vi "RGBToIntensityGraph.vi"(3 "B Array":sgl[][](array[numeric])=array200x200[40000 elements], 4 "G Array":sgl[][](array[numeric])=array200x200[40000 elements], 5 "R Array":sgl[][](array[numeric])=array200x200[40000 elements]) -> (1 "2D Picture":picture)   [LabVIEW 2015]
uses:
  <vilib>/picture/picture.llb/Draw True-Color Pixmap.vi
panel:
  out "Intensity Graph":u32[][](graph)
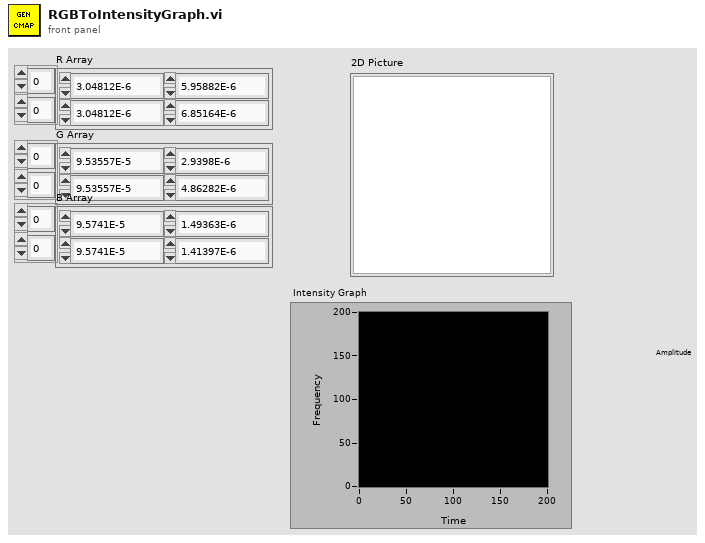
[diagram p1: front panel]
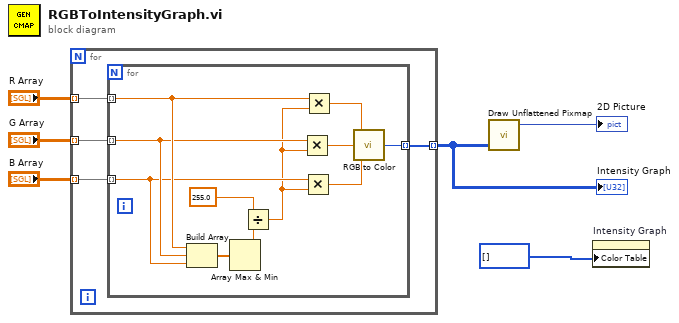
[diagram p0: block diagram]
diagram:
  n1 = for {
    tunnel: "G Array" -> [w10] mode=indexing
    tunnel: "R Array" -> [w9] mode=indexing
    tunnel: "B Array" -> [w8] mode=indexing
    tunnel: [w7] -> w1 mode=indexing
    n2 = for {
      tunnel: w10 -> [w16] mode=indexing
      tunnel: w9 -> [w17] mode=indexing
      tunnel: w8 -> [w15] mode=indexing
      tunnel: [w21] -> w7 mode=indexing
      n3 = Build Array(w17, w16, w15) -> (w19:sgl[])
      n4 = Array Max & Min(array=w19) -> (max value=w18:sgl)  [unwired: 3 out]
      n5 = Divide(x=sgl 255.0 ("max value"), y=w18) -> (x/y=w11:sgl)
      n6 = Multiply(x=w16, y=w11) -> (x*y=w13:sgl)
      n7 = Multiply(x=w15, y=w11) -> (x*y=w12:sgl)
      n8 = Multiply(x=w17, y=w11) -> (x*y=w14:sgl)
      n9 = call <vilib>:"RGB to Color.vi"("B"=w12, "G"=w13, "R"=w14) -> ("Color"=w21:u32)
    }
  }
  "Intensity Graph" <- w1
  n10 = call-poly <vilib>:"Draw Unflattened Pixmap.vi"("data (RGB format)"=w1) -> ("new picture"=→"2D Picture":picture)  [unwired: 8 in]
  n11 = property on="Intensity Graph" class="IntGraph (strict)"("Color Table"=u32[] []) -> ()  [unwired: 2 in, 2 out]
